vi "Show Panel.vi"(8 "error in (no error)":errorcluster) -> (0 "error out":errorcluster)   [LabVIEW 2015, in "Thermal Chamber Controller_DQMH.lvlib"]
doc: "Send the Show Panel request to the Module's Main.vi.\n_____\nBased on Delacor QMH Project Template 2.0.0.62.\n____\nDelacor QMH Thermal Chamber Examples 4.0.0.21\nCopyright (c) 2018, Delacor"
uses:
  Thermal Chamber Controller_DQMH.lvlib
  Show Panel Argument--cluster.ctl
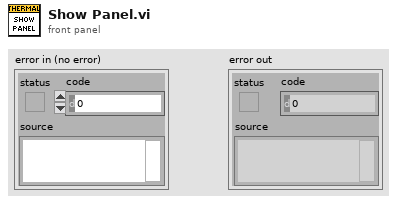
[diagram p1: front panel]
types:
  T1 = typedef "Thermal Chamber Controller_DQMH.lvlib/Request Events--cluster.ctl" = cluster{"Stop Module":refnum<user-event>, "Show Panel":refnum<user-event>, "Hide Panel":refnum<user-event>, "Get Module Execution Status":refnum<user-event>, "Show Diagram":refnum<user-event>, "Update Set Point":refnum<user-event>, "Update Ramp Rate":refnum<user-event>, "Update Heater State":refnum<user-event>, "Update Chamber Status":refnum<user-event>, "Request and Wait for Status":refnum<user-event>}
  T2 = typedef "Thermal Chamber Controller_DQMH.lvlib/Show Panel Argument--cluster.ctl" = cluster{"Show Panel?":bool}
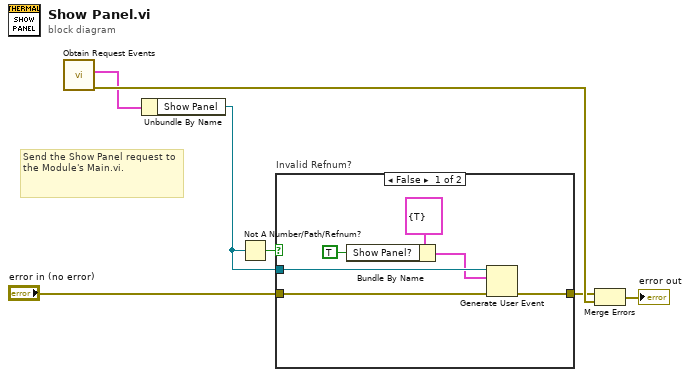
[diagram p0: block diagram]
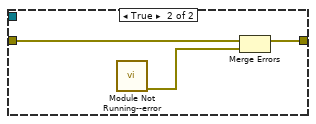
[diagram p2: hidden frame]
diagram:
  # "Send the Show Panel request to the Module's Main.vi."
  n1 = call "Obtain Request Events.vi"() -> ("error out"=w6:errorcluster, "Thermal Chamber Controller_DQMH Request Events"=w5:T1)  [unwired: 10 in]
  n2 = Unbundle By Name(w5) -> ("Show Panel"=w3:refnum<user-event>)
  n3 = Not A Number/Path/Refnum?(number/path/refnum=w3) -> (NaN/Path/Refnum?=w4:bool)
  n4 = case "Invalid Refnum?" shown="False" w4 {
    tunnel: "error in (no error)" -> [w13 w16]
    tunnel: [w12 w15] -> w1
    tunnel: w3 -> [w11 _]
    frame False {
      n5 = Bundle By Name(cluster=T2 {"Show Panel?"=TRUE} ("Show Panel Argument"), "Show Panel?"=TRUE) -> (w9:T2)
      n6 = Generate User Event(user event=w11, event data cluster=w9, error in=w13) -> (error out=w12:errorcluster)  [unwired: 1 in, 1 out]
    }
    frame True {
      n7 = call "Module Not Running--error.vi"() -> ("error out"=w14:errorcluster)  [unwired: 11 in]
      n8 = Merge Errors(w16, w14) -> (w15:errorcluster)
    }
  }
  n9 = Merge Errors(w1, w6) -> (→"error out":errorcluster)
